vi "WRP Set Property Bool.vi"(8 "error in (no error)":errorcluster, 9 "value":u8, 10 "index":i32, 11 "property":string) -> (0 "error out":errorcluster, 3 "function return":i32)   [LabVIEW 2018, in "SesWrapper.lvlib"]
doc: "int STDCALL WRP_SetPropertyBool(const String property, int index, const _bool *value);"
uses:
  SesWrapper.lvlib
  build/Debug/SESWrapper.dll
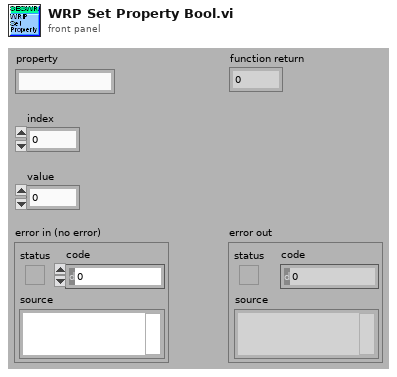
[diagram p1: front panel]
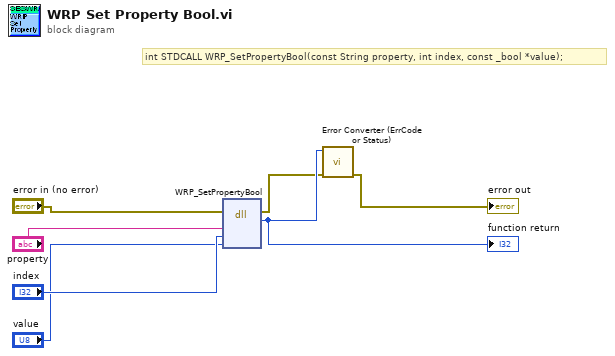
[diagram p0: block diagram]
diagram:
  # "int STDCALL WRP_SetPropertyBool(const String property, int index, const _bool *value);"
  n1 = dll-call lib="C:/Development/svn/seswrapper-lib/build/Debug/SESWrapper.*" fn="WRP_SetPropertyBool"(error in="error in (no error)", "property"="property", "index"="index", "value"="value") -> (error out=w2:errorcluster, w7:i32)  [unwired: 5 in, 1 out]
  "function return" <- w7
  n2 = call "Error Converter (ErrCode or Status).vi"("error in (no error)"=w2, "error code"=w7) -> ("error out"=→"error out":errorcluster)  [unwired: 9 in]
